vi "Get csv row data from table.vi"(8 "error in":errorcluster, 9 "Column name":string, 10 "Row (1-n)":u32=1 min=1, 11 "2D data table":string[][](array[string])) -> (0 "error out":errorcluster, 2 "Found Data?":bool, 3 "Data value":string)   [LabVIEW 2024]
panel:
  out "Columns":i32
  out "Rows without header":i32
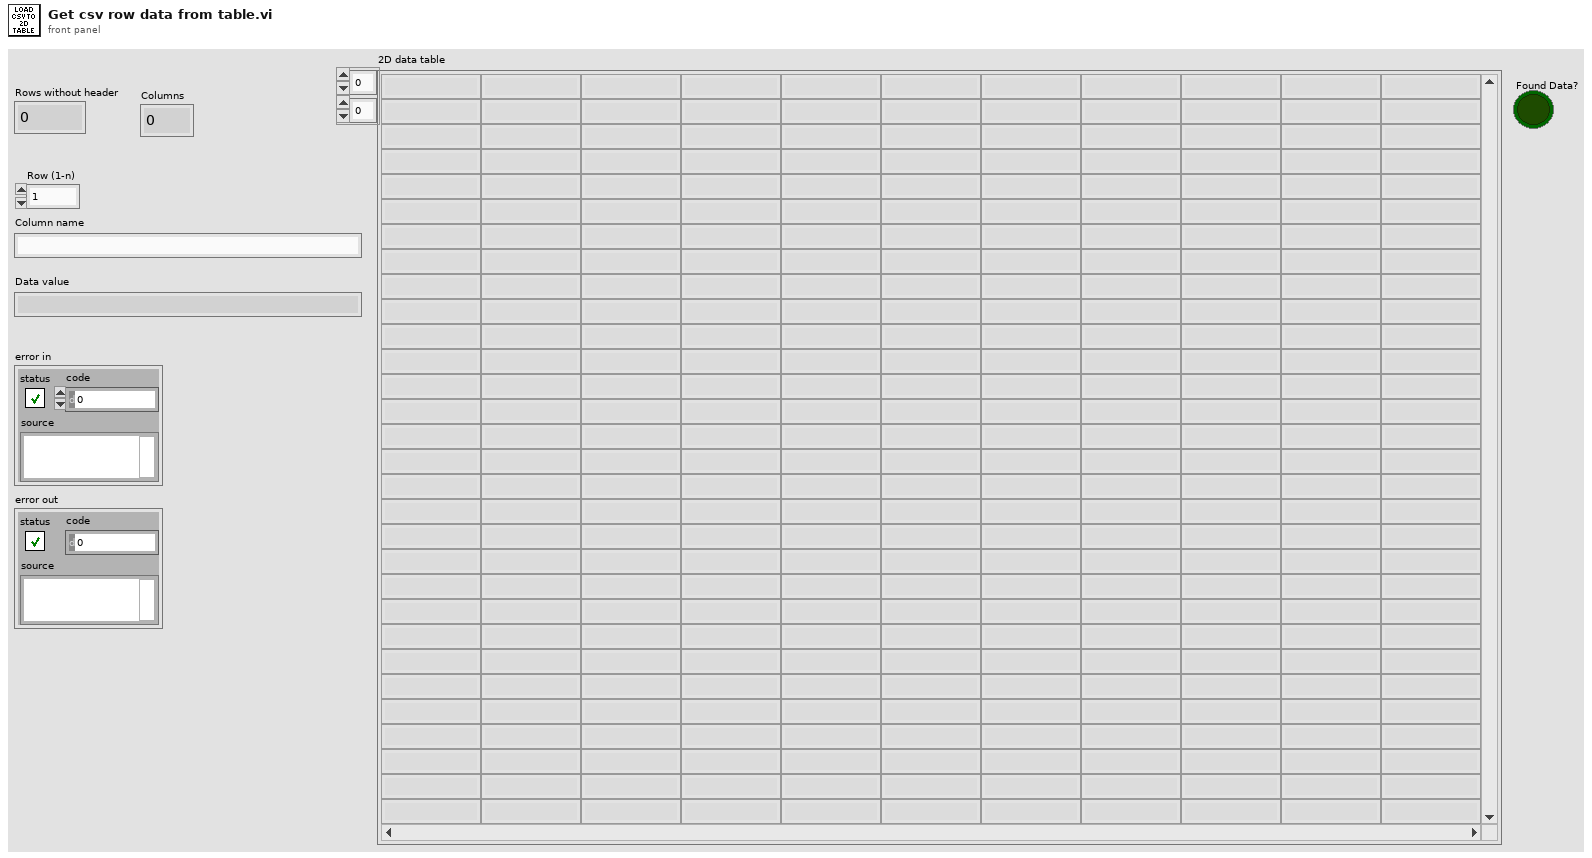
[diagram p1: front panel]
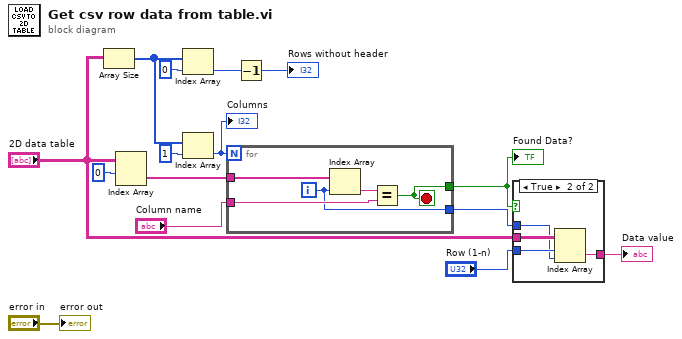
[diagram p0: block diagram]
diagram:
  n1 = Array Size(array="2D data table") -> (size(s)=w4:i32[])
  n2 = Index Array(array="2D data table", index (row)=0) -> (element=w8:string[])  [unwired: 1 in]
  n3 = Index Array(array=w4, index=0) -> (element=w2:i32)
  n4 = Index Array(array=w4, index=1) -> (element=w3:i32)
  "Columns" <- w3
  n5 = for {
    N: w3 -> [_]
    tunnel: w8 -> [w20]
    tunnel: "Column name" -> [w18]
    tunnel: [w17] -> w6
    tunnel: [w16] -> w7
    i -> [w17]
    stop <- w16 stop-if-true
    n6 = Index Array(array=w20, index=w17) -> (element=w19:string)
    n7 = Equal?(x=w19, y=w18) -> (x = y?=w16:bool)
  }
  "Found Data?" <- w7
  n8 = Decrement(x=w2) -> (x-1=→"Rows without header":i32)
  n9 = case shown="True" w7 {
    tunnel: "2D data table" -> [_ w24]
    tunnel: "Row (1-n)" -> [_ w23]
    tunnel: w6 -> [_ w22]
    tunnel: [_ w21] -> w13
    frame False {
    }
    frame True {
      n10 = Index Array(array=w24, index (row)=w23, index (col)=w22) -> (element=w21:string)
    }
  }
  "Data value" <- w13
  "error out" <- "error in"
